vi "Time_elapsed.vi"(8 "error in (no error)":errorcluster, 11 "From":timestamp) -> (0 "error out":errorcluster, 1 "Minutes":dbl, 2 "Hours":dbl, 3 "Days":dbl)   [LabVIEW 2012]
panel:
  out "Total Seconds":dbl
  out "Seconds":dbl
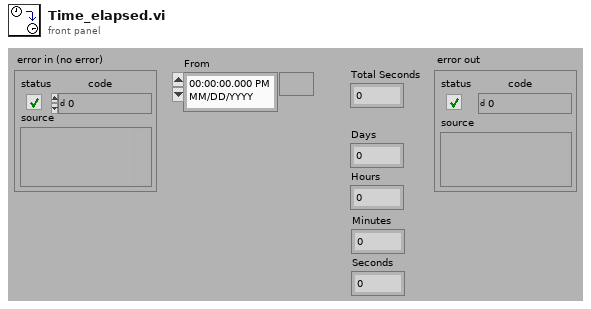
[diagram p1: front panel]
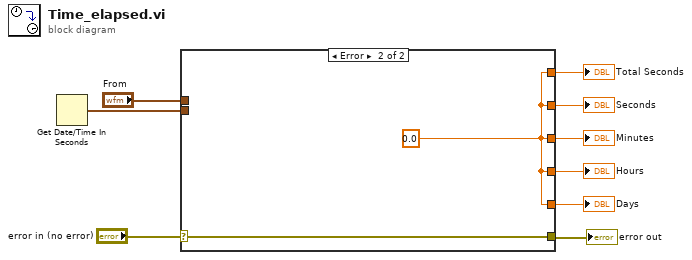
[diagram p0: block diagram]
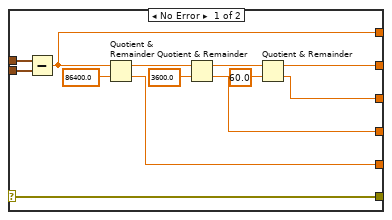
[diagram p2: hidden frame]
diagram:
  n1 = Get Date/Time In Seconds() -> (seconds since 1Jan1904=w8:timestamp)
  n2 = case shown="Error" "error in (no error)" {
    selector: "error in (no error)" -> [w15 w24]
    tunnel: "From" -> [w22 _]
    tunnel: w8 -> [w16 _]
    tunnel: [w15 w24] -> w7
    tunnel: [w14 w23] -> w5
    tunnel: [w13 w23] -> w4
    tunnel: [w12 w23] -> w3
    tunnel: [w11 w23] -> w2
    tunnel: [w10 w23] -> w1
    frame No Error {
      n3 = Subtract(x=w22, y=w16) -> (x-y=w14:dbl)
      n4 = Quotient & Remainder(x=w14, y=86400.0) -> (x-y*floor(x/y)=w19:dbl, floor(x/y)=w10:dbl)
      n5 = Quotient & Remainder(x=w19, y=3600.0) -> (x-y*floor(x/y)=w17:dbl, floor(x/y)=w11:dbl)
      n6 = Quotient & Remainder(x=w17, y=60.0) -> (x-y*floor(x/y)=w13:dbl, floor(x/y)=w12:dbl)
    }
    frame Error {
      w23 = 0.0
    }
  }
  "error out" <- w7
  "Days" <- w1
  "Hours" <- w2
  "Minutes" <- w3
  "Seconds" <- w4
  "Total Seconds" <- w5
